vi "chopdata.vi"(8 "velo":dbl[][](array[numeric]), 9 "pos":dbl[](array[numeric])) -> (1 "slam_pos":dbl[](array[numeric]))   [LabVIEW 2012]
uses:
  G_SEN.vi
  <vilib>/Analysis/baseanly.llb/Real A x B.vi
  <vilib>/Analysis/7linalg.llb/Real SVD Decomposition.vi
  <vilib>/Analysis/Matrix/Numeric/Multiply/Multiply - RM,RM.vi
  <vilib>/Analysis/baseanly.llb/A x Vector.vi
  <vilib>/Analysis/Matrix/Numeric/Conversions/Matrix To Array - RM.vi
  <vilib>/Analysis/NI_AALBase.lvlib
  <vilib>/Analysis/NI_AALPro.lvlib
  <vilib>/Analysis/Matrix/NI_Matrix.lvlib
panel:
  out "y' 2":dbl
  in  "y 2":dbl
  in  "graph":bool
  out "iter 2":i32
  out "iter":i32
  out "error":dbl
  out "R'":dbl[][](array[numeric])
  out "y'":dbl
  out "x'":dbl
  out "mindata":dbl[][](array[numeric])
  out "keydata":dbl[][](array[numeric])
  out "zero_80_240":i32[][](array[numeric])
  out "time":u32
  out "x":dbl[](array[numeric])
  out "y":dbl[](array[numeric])
  out "XY Graph":cluster{"Y":dbl[], "Y":dbl[]}[](graph)
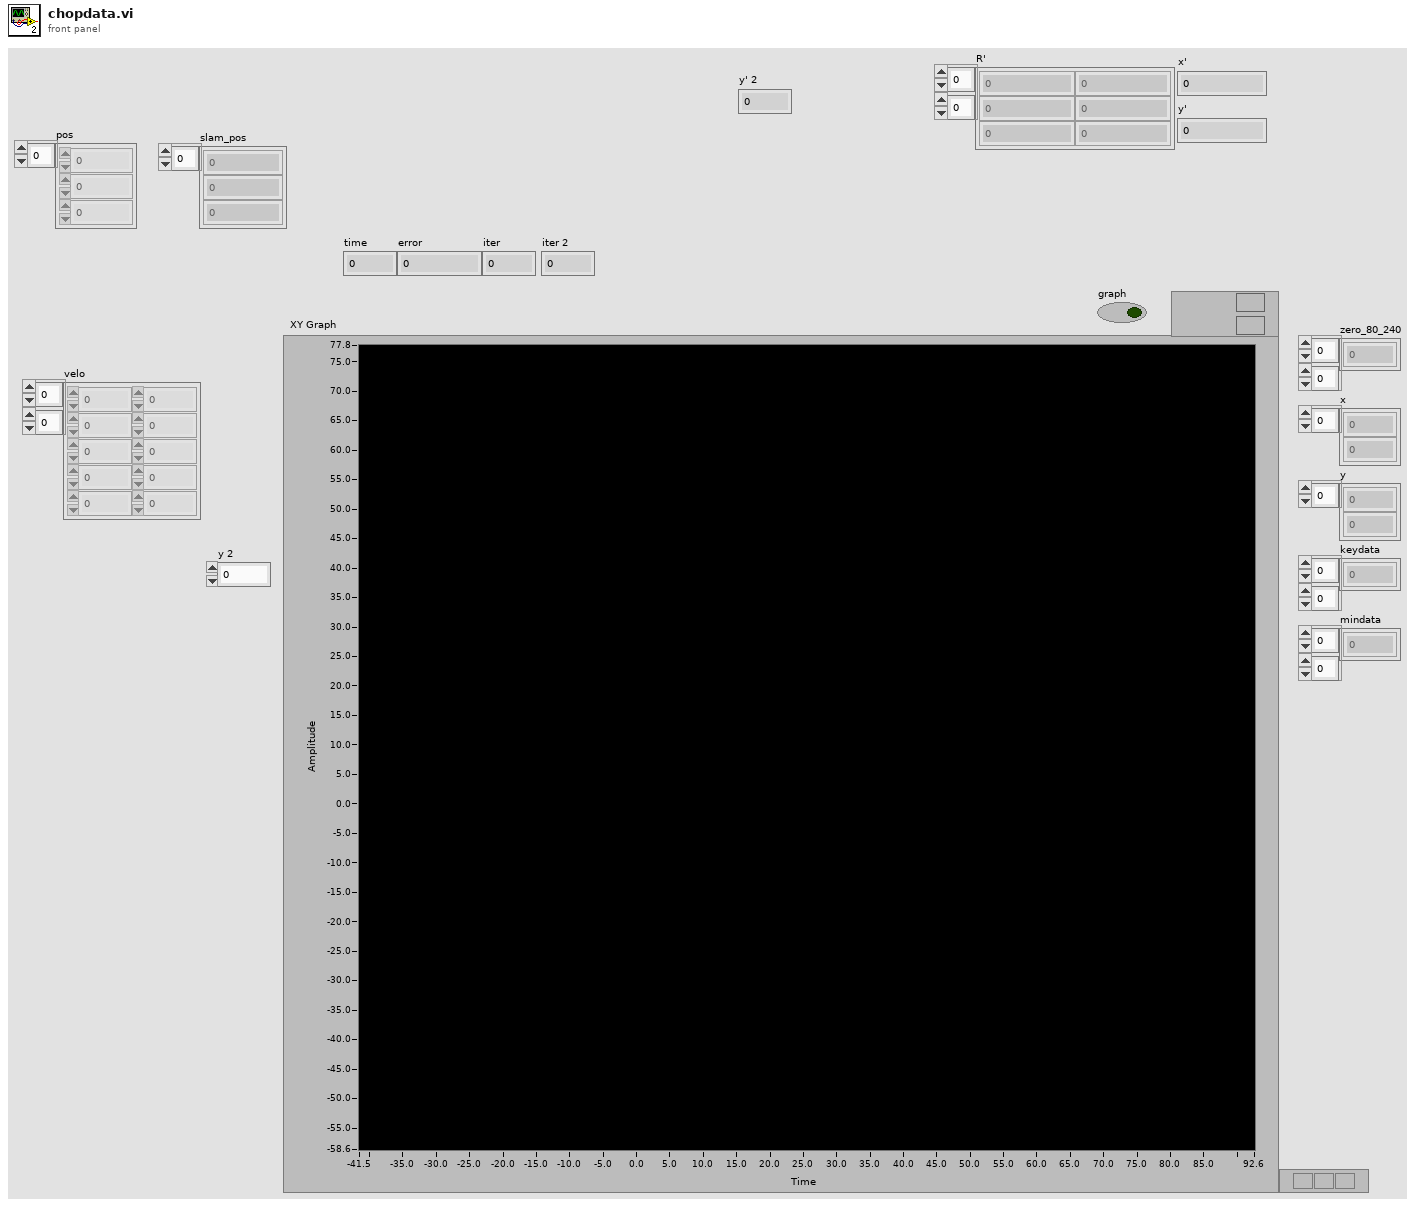
[diagram p1: front panel]
types:
  T1 = cluster{bool, "element":dbl, "element":dbl, "element":dbl}[]
  T2 = typedef "NI_Matrix.lvlib/RealMatrix.ctl" = dbl[][]
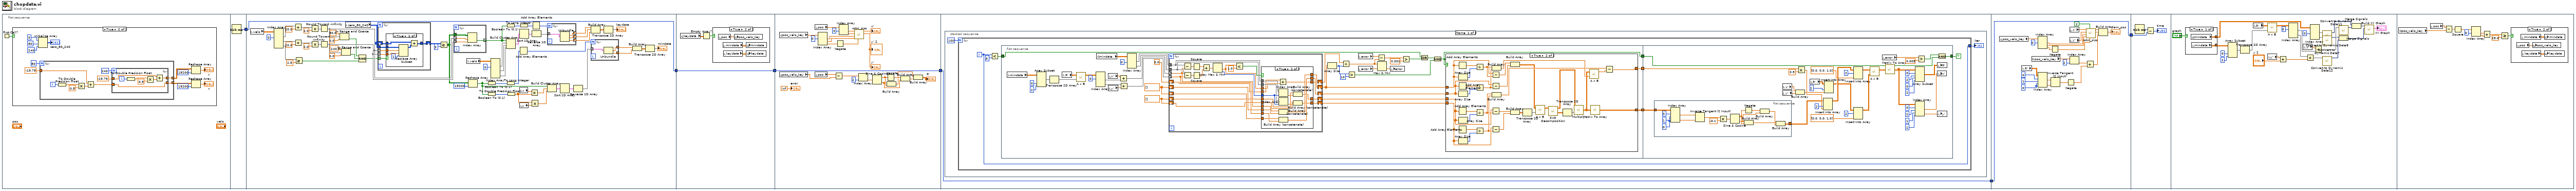
[diagram p0: block diagram]
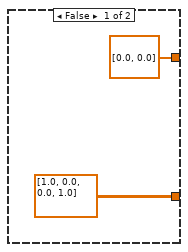
[diagram p5: hidden frame]
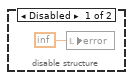
[diagram p8: hidden frame]
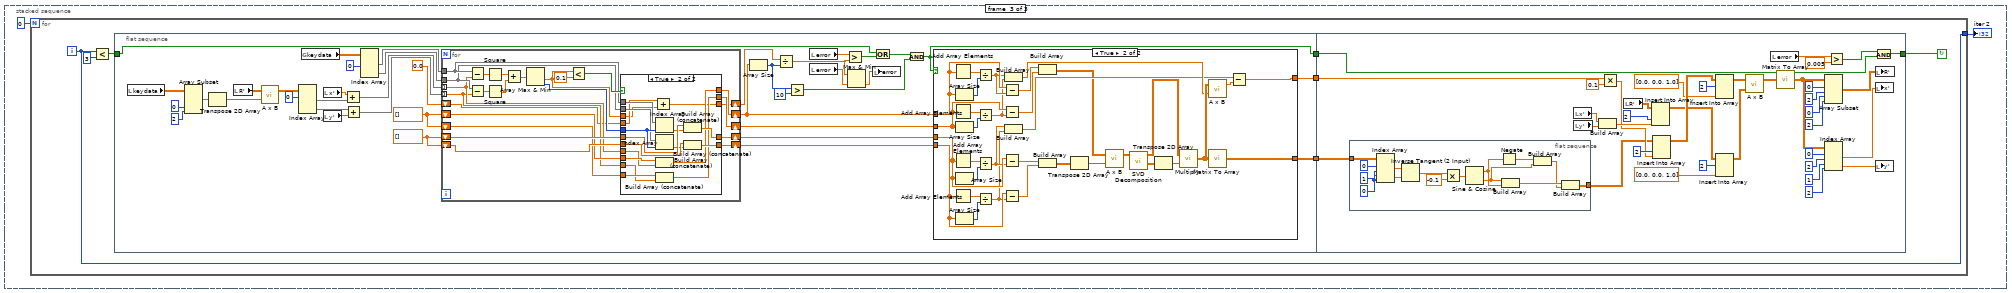
[diagram p9: hidden frame]
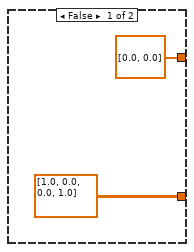
[diagram p10: hidden frame]
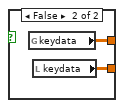
[diagram p12: hidden frame]
diagram:
  n1 = flat-sequence {
    tunnel: [w37] -> w6
    tunnel: w6 -> [w53]
    tunnel: [w53] -> w1
    tunnel: w1 -> [w129]
    tunnel: [w129] -> w5
    tunnel: w5 -> [w157]
    tunnel: [w157] -> w4
    tunnel: w4 -> [w158]
    tunnel: [w158] -> w3
    tunnel: w3 -> [w548]
    tunnel: [w548] -> w2
    tunnel: w2 -> [w550]
    frame #0 {
      n2 = First Call?() -> (First Call?: T/F=w7:bool)
      n3 = case shown="True" w7 {
        frame False {
        }
        frame True {
          n4 = Initialize Array(0, 80 ("dimension size"), 240 ("dimension size")) -> (→"zero_80_240":i32[][])
          n5 = for {
            N: 80 -> [_]
            tunnel: -19.75 -> [w27]
            tunnel: [w24] -> w12 mode=indexing
            tunnel: [w23] -> w17 mode=indexing
            i -> [w26]
            n6 = To Double Precision Float(number=w26) -> (double precision float=w22:dbl)
            n7 = Multiply(x=w22, y=0.5) -> (x*y=w20:dbl)
            n8 = Add(x=w27, y=w20) -> (x+y=w25:dbl)
            n9 = for {
              N: 240 -> [_]
              tunnel: -19.75 -> [w36]
              tunnel: [w34] -> w23 mode=indexing
              tunnel: w25 -> [w33]
              tunnel: [w33] -> w24 mode=indexing
              i -> [w35]
              n10 = To Double Precision Float(number=w35) -> (double precision float=w32:dbl)
              n11 = Multiply(x=w32, y=0.5) -> (x*y=w30:dbl)
              n12 = Add(x=w36, y=w30) -> (x+y=w34:dbl)
            }
          }
          n13 = Reshape Array(w17, 19200 ("dimension size")) -> (→"y":dbl[])
          n14 = Reshape Array(w12, 19200 ("dimension size")) -> (→"x":dbl[])
        }
      }
    }
    frame #1 {
      n15 = Tick Count (ms)() -> (millisecond timer value=w37:u32)
    }
    frame #2 {
      n16 = local read "velo"() -> (w48:dbl[][])
      n17 = Index Array(array=w48, index (col) #1=0 ("disabled index (col)")) -> (element #1=w78:dbl[], element #2=w77:dbl[], element #3=w40:dbl[])  [unwired: 5 in]
      n18 = Add(x=w78, y=20.0) -> (x+y=w74:dbl[])
      n19 = Add(x=w77, y=20.0) -> (x+y=w70:dbl[])
      n20 = Greater Or Equal?(x=w40, y=2.5) -> (x >= y?=w38:bool[])
      n21 = Multiply(x=w74, y=2.0) -> (x*y=w73:dbl[])
      n22 = Multiply(x=w70, y=2.0) -> (x*y=w69:dbl[])
      n23 = Round Toward -Infinity(1:w73) -> (0:w91:dbl[])
      n24 = Round Toward -Infinity(1:w69) -> (0:w92:dbl[])
      n25 = In Range and Coerce(upper limit=80.0, x=w91, lower limit=0.0) -> (In Range?=w86:bool[])  [unwired: 1 out]
      n26 = In Range and Coerce(upper limit=240.0, x=w92, lower limit=0.0) -> (In Range?=w87:bool[])  [unwired: 1 out]
      n27 = local read "zero_80_240"() -> (w52:i32[][])
      n28 = Compound Arithmetic op=AND(w86, w87, w38) -> (w88:bool[])
      n29 = for {
        shift-right: [w116] -> w90
        shift-left: w52 -> [w117]
        tunnel: w88 -> [w118] mode=indexing
        tunnel: w52 -> [w115]
        tunnel: w91 -> [w114] mode=indexing
        tunnel: w92 -> [w113] mode=indexing
        n30 = case shown="True" w118 {
          tunnel: w117 -> [w119 w122]
          tunnel: [w119 w120] -> w116
          tunnel: w115 -> [_ w126]
          tunnel: w114 -> [_ w125]
          tunnel: w113 -> [_ w124]
          frame False {
          }
          frame True {
            n31 = Replace Array Subset(array=w126, new element=1 ("new element/subarray"), index (row)=w125, index (col)=w124) -> (w121:i32[][])
            n32 = Add(x=w122, y=w121) -> (x+y=w120:i32[][])
          }
        }
      }
      n33 = Greater Or Equal?(x=w90, y=3) -> (x >= y?=w62:bool[][])
      n34 = for {
        tunnel: w62 -> [w112]
        tunnel: w91 -> [w111] mode=indexing
        tunnel: w92 -> [w110] mode=indexing
        tunnel: [w109] -> w95 mode=indexing
        n35 = Index Array(array=w112, index (row)=w111, index (col)=w110) -> (element=w109:bool)
      }
      n36 = local read "velo"() -> (w47:dbl[][])
      n37 = Reshape Array(w62, 19200 ("dimension size")) -> (w56:bool[])
      n38 = Boolean To (0,1)(Boolean=w56) -> (0, 1=w58:i16[])
      n39 = Boolean To (0,1)(Boolean=w56) -> (0, 1=w67:i16[])
      n40 = Index Array(array=w47, index (col) #1=0 ("disabled index (col)")) -> (element #1=w45:dbl[], element #2=w44:dbl[], element #3=w43:dbl[])  [unwired: 5 in]
      n41 = Boolean To (0,1)(Boolean=w95) -> (0, 1=w96:i16[])
      n42 = To Long Integer(number=w58) -> (32bit integer=w57:i32[])
      n43 = Build Cluster Array(w95, w45, w44, w43) -> (w93:T1)
      n44 = To Double Precision Float(number=w67) -> (double precision float=w61:dbl[])
      n45 = Add Array Elements(numeric array=w57) -> (sum=w55:i32)
      n46 = To Long Integer(number=w96) -> (32bit integer=w97:i32[])
      n47 = Sort 1D Array(array=w93) -> (sorted array=w94:T1)
      n48 = local read "x"() -> (w65:dbl[])
      n49 = local read "y"() -> (w66:dbl[])
      n50 = Multiply(x=w65, y=w61) -> (x*y=w64:dbl[])
      n51 = Multiply(x=w61, y=w66) -> (x*y=w63:dbl[])
      n52 = Add Array Elements(numeric array=w97) -> (sum=w98:i32)
      n53 = Reverse 1D Array(array=w94) -> (reversed array=w99:T1)
      n54 = for {
        N: w98 -> [_]
        tunnel: w99 -> [w108] mode=indexing
        tunnel: [w107] -> w76 mode=indexing
        tunnel: [w106] -> w75 mode=indexing
        tunnel: [w105] -> w100 mode=indexing
        n55 = Unbundle(w108) -> ("element"=w107:dbl, "element"=w106:dbl, "element"=w105:dbl)  [unwired: 1 out]
      }
      n56 = Build Cluster Array(w56, w64, w63) -> (w59:cluster{bool, dbl, dbl}[])
      n57 = Sort 1D Array(array=w59) -> (sorted array=w60:cluster{bool, dbl, dbl}[])
      n58 = Reverse 1D Array(array=w60) -> (reversed array=w54:cluster{bool, dbl, dbl}[])
      n59 = Build Array(w76, w75, w100) -> (w101:dbl[][])
      n60 = for {
        N: w55 -> [_]
        tunnel: w54 -> [w104] mode=indexing
        tunnel: [w103] -> w51 mode=indexing
        tunnel: [w102] -> w50 mode=indexing
        n61 = Unbundle(w104) -> (w103:dbl, w102:dbl)  [unwired: 1 out]
      }
      n62 = Transpose 2D Array(2D array=w101) -> (transposed array=→"keydata":dbl[][])
      n63 = Build Array(w51, w50) -> (w49:dbl[][])
      n64 = Transpose 2D Array(2D array=w49) -> (transposed array=→"mindata":dbl[][])
    }
    frame #3 {
      n65 = global read "G_SEN.vi" "keydata"() -> (w127:dbl[][])
      n66 = Empty Array?(array=w127) -> (empty?=w128:bool)
      n67 = case shown="True" w128 {
        frame False {
        }
        frame True {
          n68 = local read "pos"() -> (w130:dbl[])
          n69 = local read "mindata"() -> (w131:dbl[][])
          n70 = local read "keydata"() -> (w132:dbl[][])
          n71 = global write "G_SEN.vi" "pos_velo_key"(w130) -> ()
          n72 = global write "G_SEN.vi" "mindata"(w131) -> ()
          n73 = global write "G_SEN.vi" "keydata"(w132) -> ()
        }
      }
    }
    frame #4 {
      n74 = global read "G_SEN.vi" "pos_velo_key"() -> (w156:dbl[])
      n75 = global read "G_SEN.vi" "pos_velo_key"() -> (w143:dbl[])
      n76 = local read "pos"() -> (w150:dbl[])
      n77 = local read "pos"() -> (w144:dbl[])
      n78 = Index Array(array=w156, index #1=0 ("index")) -> (element #1=w154:dbl, element #2=w153:dbl, element #3=w152:dbl)  [unwired: 2 in]
      n79 = Subtract(x=w144, y=w143) -> (x-y=w142:dbl[])
      n80 = Negate(x=w152) -> (-x=w151:dbl)
      n81 = Index Array(array=w150, index #1=0 ("index")) -> (element #1=w148:dbl, element #2=w147:dbl)  [unwired: 1 in]
      n82 = call "rotm_siso.vi"("angle[rad]"=w151, "y0"=w153, "x0"=w154, "y"=w147, "x"=w148) -> ("y'"=→"y'" →"y' 2":dbl, "x'"=→"x'":dbl)  [unwired: 5 in]
      n83 = Index Array(array=w142, index=2) -> (element=w133:dbl)
      n84 = Sine & Cosine(0:w133) -> (1:w140:dbl, 2:w138:dbl)
      n85 = Negate(x=w140) -> (-x=w139:dbl)
      n86 = Build Array(w138, w140) -> (w137:dbl[])
      n87 = Build Array(w139, w138) -> (w136:dbl[])
      n88 = Build Array(w137, w136) -> (→"R'":dbl[][])
      "error" <- inf
    }
    frame #5 {
      n89 = stacked-sequence {
        frame #0 {
          n90 = for {
            N: 100 -> [_]
            tunnel: [w164] -> w159
            i -> [w164]
            stop <- w161 continue-if-true
            n91 = Less?(x=w164, y=3) -> (x < y?=w162:bool)
            n92 = flat-sequence {
              tunnel: [w208] -> w167
              tunnel: [w207] -> w166
              tunnel: [w206] -> w165
              tunnel: w162 -> [w205]
              tunnel: w167 -> [w292]
              tunnel: w166 -> [w296]
              tunnel: w165 -> [w297]
              tunnel: [w291] -> w161
              frame #0 {
                w185 = dbl[] []
                w186 = dbl[] []
                n93 = local read "mindata"() -> (w202:dbl[][])
                n94 = Array Subset(array=w202, index (col)=0 ("index"), length (col)=2 ("length")) -> (w199:dbl[][])  [unwired: 2 in]
                n95 = Transpose 2D Array(2D array=w199) -> (transposed array=w190:dbl[][])
                n96 = local read "R'"() -> (w191:dbl[][])
                n97 = call-poly <vilib>:"A x B.vi"("B"=w190, "A"=w191) -> ("A x B"=w189:T2)  [unwired: 1 out]
                n98 = Index Array(array=w189, index (row) #1=0 ("index (row)")) -> (element #1=w188:dbl[], element #2=w187:dbl[])  [unwired: 3 in]
                n99 = global read "G_SEN.vi" "mindata"() -> (w197:dbl[][])
                n100 = local read "x'"() -> (w204:dbl)
                n101 = local read "y'"() -> (w203:dbl)
                n102 = Add(x=w204, y=w188) -> (x+y=w193:dbl[])
                n103 = Add(x=w187, y=w203) -> (x+y=w192:dbl[])
                n104 = Index Array(array=w197, index (col) #1=0 ("disabled index (col)")) -> (element #1=w195:dbl[], element #2=w194:dbl[])  [unwired: 3 in]
                n105 = for {
                  tunnel: w195 -> [w259]
                  tunnel: w194 -> [w254]
                  tunnel: w193 -> [w249] mode=indexing
                  tunnel: w192 -> [w248] mode=indexing
                  shift-right: [w257] -> w180
                  shift-left: w186 -> [w260]
                  shift-right: [w255] -> w184
                  shift-left: w186 -> [w256]
                  shift-right: [w252] -> w176
                  shift-left: w185 -> [w253]
                  shift-right: [w250] -> w182
                  shift-left: w185 -> [w251]
                  shift-right: [w245] -> w179
                  shift-left: 0.0 -> [w247]
                  n106 = Subtract(x=w259, y=w249) -> (x-y=w266:dbl[])
                  n107 = Subtract(x=w254, y=w248) -> (x-y=w265:dbl[])
                  n108 = Square(x=w266) -> (x^2=w264:dbl[])
                  n109 = Square(x=w265) -> (x^2=w263:dbl[])
                  n110 = Add(x=w264, y=w263) -> (x+y=w262:dbl[])
                  n111 = Array Max & Min(array=w262) -> (min value=w246:dbl, min index (indices)=w258:i32)  [unwired: 2 out]
                  n112 = Less?(x=w246, y=1.0) -> (x < y?=w261:bool)
                  n113 = case shown="True" w261 {
                    tunnel: w260 -> [w271 w289]
                    tunnel: w259 -> [_ w288]
                    tunnel: w258 -> [_ w283]
                    tunnel: [w271 w286] -> w257
                    tunnel: w256 -> [w270 w285]
                    tunnel: [w270 w284] -> w255
                    tunnel: w254 -> [_ w282]
                    tunnel: w253 -> [w268 w280]
                    tunnel: [w268 w279] -> w252
                    tunnel: w251 -> [w269 w278]
                    tunnel: [w269 w277] -> w250
                    tunnel: w249 -> [_ w276]
                    tunnel: w248 -> [_ w275]
                    tunnel: w247 -> [w267 w274]
                    tunnel: w246 -> [_ w273]
                    tunnel: [w267 w272] -> w245
                    frame False {
                    }
                    frame True {
                      n114 = Add(x=w274, y=w273) -> (x+y=w272:dbl)
                      n115 = Index Array(array=w288, index=w283) -> (element=w287:dbl)
                      n116 = Index Array(array=w282, index=w283) -> (element=w281:dbl)
                      n117 = Build Array (concatenate)(w280, w276) -> (w279:dbl[])
                      n118 = Build Array (concatenate)(w278, w275) -> (w277:dbl[])
                      n119 = Build Array (concatenate)(w289, w287) -> (w286:dbl[])
                      n120 = Build Array (concatenate)(w285, w281) -> (w284:dbl[])
                    }
                  }
                }
                n121 = Array Size(array=w176) -> (size(s)=w178:i32)
                n122 = Divide(x=w179, y=w178) -> (x/y=w171:dbl)
                n123 = Greater?(x=w178, y=10) -> (0:w175:bool)
                n124 = local read "error"() -> (w172:dbl)
                n125 = local read "error"() -> (w177:dbl)
                n126 = Subtract(x=w172, y=w171) -> (x-y=w170:dbl)
                n127 = Max & Min(x=w171, y=w177) -> (min(x,y)=w173:dbl)  [unwired: 1 out]
                n128 = local write "error"(w173) -> ()
                n129 = Greater?(x=w170, y=0.001) -> (0:w169:bool)
                n130 = Or(x=w205, y=w169) -> (x .or. y?=w174:bool)
                n131 = And(x=w174, y=w175) -> (x .and. y?=w208:bool)
                n132 = case shown="True" w208 {
                  tunnel: [dbl[][] [[1.0, 0.0], [0.0, 1.0]] w240] -> w207
                  tunnel: w180 -> [_ w236]
                  tunnel: w184 -> [_ w232]
                  tunnel: w182 -> [_ w228]
                  tunnel: w176 -> [_ w224]
                  tunnel: [dbl[] [0.0, 0.0] w214] -> w206
                  frame False {
                  }
                  frame True {
                    n133 = Add Array Elements(numeric array=w224) -> (sum=w225:dbl)
                    n134 = Add Array Elements(numeric array=w228) -> (sum=w230:dbl)
                    n135 = Add Array Elements(numeric array=w236) -> (sum=w238:dbl)
                    n136 = Add Array Elements(numeric array=w232) -> (sum=w233:dbl)
                    n137 = Array Size(array=w224) -> (size(s)=w226:i32)
                    n138 = Array Size(array=w228) -> (size(s)=w229:i32)
                    n139 = Array Size(array=w236) -> (size(s)=w237:i32)
                    n140 = Array Size(array=w232) -> (size(s)=w234:i32)
                    n141 = Divide(x=w225, y=w226) -> (x/y=w222:dbl)
                    n142 = Divide(x=w230, y=w229) -> (x/y=w221:dbl)
                    n143 = Divide(x=w238, y=w237) -> (x/y=w220:dbl)
                    n144 = Divide(x=w233, y=w234) -> (x/y=w219:dbl)
                    n145 = Subtract(x=w224, y=w222) -> (x-y=w223:dbl[])
                    n146 = Subtract(x=w228, y=w221) -> (x-y=w227:dbl[])
                    n147 = Subtract(x=w236, y=w220) -> (x-y=w235:dbl[])
                    n148 = Subtract(x=w232, y=w219) -> (x-y=w231:dbl[])
                    n149 = Build Array(w222, w221) -> (w217:dbl[])
                    n150 = Build Array(w220, w219) -> (w215:dbl[])
                    n151 = Build Array(w223, w227) -> (w211:dbl[][])
                    n152 = Build Array(w235, w231) -> (w213:dbl[][])
                    n153 = Transpose 2D Array(2D array=w213) -> (transposed array=w212:dbl[][])
                    n154 = call-poly <vilib>:"A x B.vi"("B"=w212, "A"=w211) -> ("A x B"=w239:T2)  [unwired: 1 out]
                    n155 = call-poly <vilib>:"SVD Decomposition.vi"("A"=w239) -> ("Matrix V"=w241:T2, "Matrix U"=w242:T2)  [unwired: 6 in, 3 out]
                    n156 = Transpose 2D Array(2D array=w241) -> (transposed array=w243:T2)
                    n157 = call-poly <vilib>:"Multiply.vi"("Real Matrix B"=w243, "Real Matrix A"=w242) -> ("A * B"=w218:T2)
                    n158 = call-poly <vilib>:"A x B.vi"("Vector"=w217, "A"=w218) -> ("A x Vector"=w216:dbl[])  [unwired: 1 out]
                    n159 = call-poly <vilib>:"Matrix To Array.vi"("Real Matrix"=w218) -> ("Real 2D Array"=w240:dbl[][])
                    n160 = Subtract(x=w215, y=w216) -> (x-y=w214:dbl[])
                  }
                }
              }
              frame #1 {
                n161 = flat-sequence {
                  tunnel: w296 -> [w336]
                  tunnel: [w327] -> w295
                  frame #0 {
                    w341 = 0 ("disabled index (col)")
                    n162 = Index Array(array=w336, index (row) #1=0 ("disabled index (row)"), index (col) #1=1 ("disabled index (col)"), index (row) #2=w341, index (col) #2=w341) -> (element #1=w337:dbl, element #2=w338:dbl)
                    n163 = Inverse Tangent (2 Input)(1:w338, 2:w337) -> (0:w335:dbl)
                    n164 = Multiply(x=w335, y=-0.1) -> (x*y=w328:dbl)
                    n165 = Sine & Cosine(0:w328) -> (1:w333:dbl, 2:w331:dbl)
                    n166 = Negate(x=w333) -> (-x=w332:dbl)
                    n167 = Build Array(w331, w333) -> (w330:dbl[])
                    n168 = Build Array(w332, w331) -> (w329:dbl[])
                    n169 = Build Array(w330, w329) -> (w327:dbl[][])
                  }
                }
                n170 = local read "x'"() -> (w316:dbl)
                n171 = local read "y'"() -> (w317:dbl)
                n172 = Build Array(w316, w317) -> (w315:dbl[])
                n173 = Multiply(x=w297, y=0.5) -> (x*y=w299:dbl[])
                n174 = local read "R'"() -> (w319:dbl[][])
                n175 = Insert Into Array(array=w295, index (col)=2 ("disabled index (col)"), new element=w299) -> (w325:dbl[][])  [unwired: 1 in]
                n176 = Insert Into Array(array=w319, index (col)=2 ("disabled index (col)"), new element=w315) -> (w320:dbl[][])  [unwired: 1 in]
                n177 = Insert Into Array(array=w325, index (row)=2, new element=dbl[] [0.0, 0.0, 1.0]) -> (w314:dbl[][])  [unwired: 1 in]
                n178 = Insert Into Array(array=w320, index (row)=2, new element=dbl[] [0.0, 0.0, 1.0]) -> (w313:dbl[][])  [unwired: 1 in]
                n179 = call-poly <vilib>:"A x B.vi"("B"=w313, "A"=w314) -> ("A x B"=w308:T2)  [unwired: 1 out]
                n180 = local read "error"() -> (w290:dbl)
                n181 = call-poly <vilib>:"Matrix To Array.vi"("Real Matrix"=w308) -> ("Real 2D Array"=w306:dbl[][])
                n182 = Array Subset(array=w306, index (row)=0 ("index"), length (row)=2 ("length"), index (col)=0 ("index"), length (col)=2 ("length")) -> (w307:dbl[][])
                n183 = Index Array(array=w306, index (row) #1=0 ("disabled index (row)"), index (col) #1=2 ("disabled index (col)"), index (row) #2=1 ("index (row)"), index (col) #2=2 ("disabled index (col)")) -> (element #1=w301:dbl, element #2=w300:dbl)
                n184 = Greater?(x=w290, y=0.005) -> (0:w293:bool)
                n185 = And(x=w293, y=w292) -> (x .and. y?=w291:bool)
                n186 = local write "R'"(w307) -> ()
                n187 = local write "x'"(w301) -> ()
                n188 = local write "y'"(w300) -> ()
              }
            }
          }
          "iter" <- w159
        }
        frame #1 {
          n189 = disable-structure shown="Enabled" {
            frame Disabled {
              n190 = local write "error"(inf) -> ()
            }
            frame Enabled {
            }
          }
        }
        frame #2 {
          n191 = for {
            N: 0 -> [_]
            tunnel: [w348] -> w343
            i -> [w348]
            stop <- w345 continue-if-true
            n192 = Less?(x=w348, y=3) -> (x < y?=w346:bool)
            n193 = flat-sequence {
              tunnel: [w390] -> w351
              tunnel: [w389] -> w350
              tunnel: [w388] -> w349
              tunnel: w346 -> [w387]
              tunnel: w351 -> [w473]
              tunnel: w350 -> [w478]
              tunnel: w349 -> [w479]
              tunnel: [w472] -> w345
              frame #0 {
                w367 = dbl[] []
                w368 = dbl[] []
                n194 = local read "keydata"() -> (w384:dbl[][])
                n195 = Array Subset(array=w384, index (col)=0 ("index"), length (col)=2 ("length")) -> (w381:dbl[][])  [unwired: 2 in]
                n196 = Transpose 2D Array(2D array=w381) -> (transposed array=w372:dbl[][])
                n197 = local read "R'"() -> (w373:dbl[][])
                n198 = call-poly <vilib>:"A x B.vi"("B"=w372, "A"=w373) -> ("A x B"=w371:T2)  [unwired: 1 out]
                n199 = Index Array(array=w371, index (row) #1=0 ("index (row)")) -> (element #1=w370:dbl[], element #2=w369:dbl[])  [unwired: 3 in]
                n200 = global read "G_SEN.vi" "keydata"() -> (w379:dbl[][])
                n201 = local read "x'"() -> (w386:dbl)
                n202 = local read "y'"() -> (w385:dbl)
                n203 = Add(x=w386, y=w370) -> (x+y=w375:dbl[])
                n204 = Add(x=w369, y=w385) -> (x+y=w374:dbl[])
                n205 = Index Array(array=w379, index (col) #1=0 ("disabled index (col)")) -> (element #1=w377:dbl[], element #2=w376:dbl[])  [unwired: 3 in]
                n206 = for {
                  tunnel: w377 -> [w441]
                  tunnel: w376 -> [w436]
                  tunnel: w375 -> [w431] mode=indexing
                  tunnel: w374 -> [w430] mode=indexing
                  shift-right: [w439] -> w361
                  shift-left: w368 -> [w442]
                  shift-right: [w437] -> w366
                  shift-left: w368 -> [w438]
                  shift-right: [w434] -> w355
                  shift-left: w367 -> [w435]
                  shift-right: [w432] -> w363
                  shift-left: w367 -> [w433]
                  shift-right: [w427] -> w360
                  shift-left: 0.0 -> [w429]
                  n207 = Subtract(x=w441, y=w431) -> (x-y=w448:dbl[])
                  n208 = Subtract(x=w436, y=w430) -> (x-y=w447:dbl[])
                  n209 = Square(x=w448) -> (x^2=w446:dbl[])
                  n210 = Square(x=w447) -> (x^2=w445:dbl[])
                  n211 = Add(x=w446, y=w445) -> (x+y=w444:dbl[])
                  n212 = Array Max & Min(array=w444) -> (min value=w428:dbl, min index (indices)=w440:i32)  [unwired: 2 out]
                  n213 = Less?(x=w428, y=0.1) -> (x < y?=w443:bool)
                  n214 = case shown="True" w443 {
                    tunnel: w442 -> [w453 w471]
                    tunnel: w441 -> [_ w470]
                    tunnel: w440 -> [_ w465]
                    tunnel: [w453 w468] -> w439
                    tunnel: w438 -> [w452 w467]
                    tunnel: [w452 w466] -> w437
                    tunnel: w436 -> [_ w464]
                    tunnel: w435 -> [w450 w462]
                    tunnel: [w450 w461] -> w434
                    tunnel: w433 -> [w451 w460]
                    tunnel: [w451 w459] -> w432
                    tunnel: w431 -> [_ w458]
                    tunnel: w430 -> [_ w457]
                    tunnel: w429 -> [w449 w456]
                    tunnel: w428 -> [_ w455]
                    tunnel: [w449 w454] -> w427
                    frame False {
                    }
                    frame True {
                      n215 = Add(x=w456, y=w455) -> (x+y=w454:dbl)
                      n216 = Index Array(array=w470, index=w465) -> (element=w469:dbl)
                      n217 = Index Array(array=w464, index=w465) -> (element=w463:dbl)
                      n218 = Build Array (concatenate)(w462, w458) -> (w461:dbl[])
                      n219 = Build Array (concatenate)(w460, w457) -> (w459:dbl[])
                      n220 = Build Array (concatenate)(w471, w469) -> (w468:dbl[])
                      n221 = Build Array (concatenate)(w467, w463) -> (w466:dbl[])
                    }
                  }
                }
                n222 = Array Size(array=w355) -> (size(s)=w359:i32)
                n223 = Divide(x=w360, y=w359) -> (x/y=w358:dbl)
                n224 = Greater?(x=w359, y=10) -> (0:w353:bool)
                n225 = local read "error"() -> (w364:dbl)
                n226 = local read "error"() -> (w357:dbl)
                n227 = Greater?(x=w364, y=w358) -> (0:w354:bool)
                n228 = Max & Min(x=w358, y=w357) -> (min(x,y)=w356:dbl)  [unwired: 1 out]
                n229 = local write "error"(w356) -> ()
                n230 = Or(x=w387, y=w354) -> (x .or. y?=w352:bool)
                n231 = And(x=w352, y=w353) -> (x .and. y?=w390:bool)
                n232 = case shown="True" w390 {
                  tunnel: [dbl[][] [[1.0, 0.0], [0.0, 1.0]] w422] -> w389
                  tunnel: w361 -> [_ w418]
                  tunnel: w366 -> [_ w414]
                  tunnel: w363 -> [_ w410]
                  tunnel: w355 -> [_ w406]
                  tunnel: [dbl[] [0.0, 0.0] w396] -> w388
                  frame False {
                  }
                  frame True {
                    n233 = Add Array Elements(numeric array=w406) -> (sum=w407:dbl)
                    n234 = Add Array Elements(numeric array=w410) -> (sum=w412:dbl)
                    n235 = Add Array Elements(numeric array=w418) -> (sum=w420:dbl)
                    n236 = Add Array Elements(numeric array=w414) -> (sum=w415:dbl)
                    n237 = Array Size(array=w406) -> (size(s)=w408:i32)
                    n238 = Array Size(array=w410) -> (size(s)=w411:i32)
                    n239 = Array Size(array=w418) -> (size(s)=w419:i32)
                    n240 = Array Size(array=w414) -> (size(s)=w416:i32)
                    n241 = Divide(x=w407, y=w408) -> (x/y=w404:dbl)
                    n242 = Divide(x=w412, y=w411) -> (x/y=w403:dbl)
                    n243 = Divide(x=w420, y=w419) -> (x/y=w402:dbl)
                    n244 = Divide(x=w415, y=w416) -> (x/y=w401:dbl)
                    n245 = Subtract(x=w406, y=w404) -> (x-y=w405:dbl[])
                    n246 = Subtract(x=w410, y=w403) -> (x-y=w409:dbl[])
                    n247 = Subtract(x=w418, y=w402) -> (x-y=w417:dbl[])
                    n248 = Subtract(x=w414, y=w401) -> (x-y=w413:dbl[])
                    n249 = Build Array(w404, w403) -> (w399:dbl[])
                    n250 = Build Array(w402, w401) -> (w397:dbl[])
                    n251 = Build Array(w405, w409) -> (w393:dbl[][])
                    n252 = Build Array(w417, w413) -> (w395:dbl[][])
                    n253 = Transpose 2D Array(2D array=w395) -> (transposed array=w394:dbl[][])
                    n254 = call-poly <vilib>:"A x B.vi"("B"=w394, "A"=w393) -> ("A x B"=w421:T2)  [unwired: 1 out]
                    n255 = call-poly <vilib>:"SVD Decomposition.vi"("A"=w421) -> ("Matrix V"=w423:T2, "Matrix U"=w424:T2)  [unwired: 6 in, 3 out]
                    n256 = Transpose 2D Array(2D array=w423) -> (transposed array=w425:T2)
                    n257 = call-poly <vilib>:"Multiply.vi"("Real Matrix B"=w425, "Real Matrix A"=w424) -> ("A * B"=w400:T2)
                    n258 = call-poly <vilib>:"A x B.vi"("Vector"=w399, "A"=w400) -> ("A x Vector"=w398:dbl[])  [unwired: 1 out]
                    n259 = call-poly <vilib>:"Matrix To Array.vi"("Real Matrix"=w400) -> ("Real 2D Array"=w422:dbl[][])
                    n260 = Subtract(x=w397, y=w398) -> (x-y=w396:dbl[])
                  }
                }
              }
              frame #1 {
                n261 = flat-sequence {
                  tunnel: w478 -> [w518]
                  tunnel: [w509] -> w477
                  frame #0 {
                    w523 = 0 ("disabled index (col)")
                    n262 = Index Array(array=w518, index (row) #1=0 ("disabled index (row)"), index (col) #1=1 ("disabled index (col)"), index (row) #2=w523, index (col) #2=w523) -> (element #1=w519:dbl, element #2=w520:dbl)
                    n263 = Inverse Tangent (2 Input)(1:w520, 2:w519) -> (0:w517:dbl)
                    n264 = Multiply(x=w517, y=-0.1) -> (x*y=w510:dbl)
                    n265 = Sine & Cosine(0:w510) -> (1:w515:dbl, 2:w513:dbl)
                    n266 = Negate(x=w515) -> (-x=w514:dbl)
                    n267 = Build Array(w513, w515) -> (w512:dbl[])
                    n268 = Build Array(w514, w513) -> (w511:dbl[])
                    n269 = Build Array(w512, w511) -> (w509:dbl[][])
                  }
                }
                n270 = local read "x'"() -> (w498:dbl)
                n271 = local read "y'"() -> (w499:dbl)
                n272 = Build Array(w498, w499) -> (w497:dbl[])
                n273 = Multiply(x=w479, y=0.1) -> (x*y=w481:dbl[])
                n274 = local read "R'"() -> (w501:dbl[][])
                n275 = Insert Into Array(array=w501, index (col)=2 ("disabled index (col)"), new element=w497) -> (w502:dbl[][])  [unwired: 1 in]
                n276 = Insert Into Array(array=w477, index (col)=2 ("disabled index (col)"), new element=w481) -> (w507:dbl[][])  [unwired: 1 in]
                n277 = Insert Into Array(array=w507, index (row)=2, new element=dbl[] [0.0, 0.0, 1.0]) -> (w496:dbl[][])  [unwired: 1 in]
                n278 = Insert Into Array(array=w502, index (row)=2, new element=dbl[] [0.0, 0.0, 1.0]) -> (w495:dbl[][])  [unwired: 1 in]
                n279 = call-poly <vilib>:"A x B.vi"("B"=w495, "A"=w496) -> ("A x B"=w490:T2)  [unwired: 1 out]
                n280 = local read "error"() -> (w475:dbl)
                n281 = call-poly <vilib>:"Matrix To Array.vi"("Real Matrix"=w490) -> ("Real 2D Array"=w488:dbl[][])
                n282 = Array Subset(array=w488, index (row)=0 ("index"), length (row)=2 ("length"), index (col)=0 ("index"), length (col)=2 ("length")) -> (w489:dbl[][])
                n283 = Index Array(array=w488, index (row) #1=0 ("disabled index (row)"), index (col) #1=2 ("disabled index (col)"), index (row) #2=1 ("index (row)"), index (col) #2=2 ("disabled index (col)")) -> (element #1=w483:dbl, element #2=w482:dbl)
                n284 = Greater?(x=w475, y=0.005) -> (0:w474:bool)
                n285 = And(x=w474, y=w473) -> (x .and. y?=w472:bool)
                n286 = local write "R'"(w489) -> ()
                n287 = local write "x'"(w483) -> ()
                n288 = local write "y'"(w482) -> ()
              }
            }
          }
          "iter 2" <- w343
        }
      }
    }
    frame #6 {
      w543 = 0 ("disabled index (col)")
      n289 = global read "G_SEN.vi" "pos_velo_key"() -> (w538:dbl[])
      n290 = local read "R'"() -> (w542:dbl[][])
      n291 = global read "G_SEN.vi" "pos_velo_key"() -> (w541:dbl[])
      n292 = Index Array(array=w538, index #1=0 ("index")) -> (element #1=w536:dbl, element #2=w535:dbl, element #3=w534:dbl)  [unwired: 2 in]
      n293 = Index Array(array=w542, index (row) #1=0 ("disabled index (row)"), index (col) #1=1 ("disabled index (col)"), index (row) #2=w543, index (col) #2=w543) -> (element #1=w547:dbl, element #2=w546:dbl)
      n294 = Negate(x=w534) -> (-x=w533:dbl)
      n295 = Inverse Tangent (2 Input)(1:w546, 2:w547) -> (0:w525:dbl)
      n296 = Negate(x=w525) -> (-x=w524:dbl)
      n297 = local read "x'"() -> (w532:dbl)
      n298 = local read "y'"() -> (w531:dbl)
      n299 = Index Array(array=w541, index=2) -> (element=w539:dbl)
      n300 = Add(x=w539, y=w524) -> (x+y=w527:dbl)
      n301 = call "rotm_siso.vi"("angle[rad]"=w533, "reverse"=TRUE, "y0"=w535, "x0"=w536, "y"=w531, "x"=w532) -> ("y'"=w528:dbl, "x'"=w529:dbl)  [unwired: 4 in]
      n302 = Build Array(w529, w528, w527) -> (→"slam_pos":dbl[])
    }
    frame #7 {
      n303 = Tick Count (ms)() -> (millisecond timer value=w551:u32)
      n304 = Subtract(x=w551, y=w550) -> (x-y=→"time":u32)
    }
    frame #8 {
      n305 = case shown="True" "graph" {
        tunnel: [w581 w583] -> w575
        tunnel: [w580 w582] -> w568
        frame True {
          n306 = global read "G_SEN.vi" "mindata"() -> (w581:dbl[][])
          n307 = local read "mindata"() -> (w580:dbl[][])
        }
        frame False {
          n308 = global read "G_SEN.vi" "keydata"() -> (w583:dbl[][])
          n309 = local read "keydata"() -> (w582:dbl[][])
        }
      }
      n310 = Array Subset(array=w568, index (col)=0 ("index"), length (col)=2 ("length")) -> (w565:dbl[][])  [unwired: 2 in]
      n311 = Transpose 2D Array(2D array=w565) -> (transposed array=w564:dbl[][])
      n312 = local read "R'"() -> (w569:dbl[][])
      n313 = call-poly <vilib>:"A x B.vi"("B"=w564, "A"=w569) -> ("A x B"=w563:T2)  [unwired: 1 out]
      n314 = local read "y'"() -> (w554:dbl)
      n315 = Add(x=w554, y="y 2") -> (x+y=w553:dbl)
      n316 = Index Array(array=w563, index (row) #1=0 ("index (row)")) -> (element #1=w573:dbl[], element #2=w572:dbl[])  [unwired: 3 in]
      n317 = local read "x'"() -> (w574:dbl)
      n318 = Add(x=w572, y=w553) -> (x+y=w570:dbl[])
      n319 = Index Array(array=w575, index (col) #1=0 ("disabled index (col)")) -> (element #1=w577:dbl[], element #2=w578:dbl[])  [unwired: 3 in]
      n320 = Add(x=w574, y=w573) -> (x+y=w571:dbl[])
      n321 = call "Convert to Dynamic Data8"("Array"=w577) -> ("Dynamic Data Type"=w561:dynamicdata)  [unwired: 3 in]
      n322 = call "Convert to Dynamic Data7"("Array"=w578) -> ("Dynamic Data Type"=w558:dynamicdata)  [unwired: 3 in]
      n323 = call "Convert to Dynamic Data12"("Array"=w570) -> ("Dynamic Data Type"=w556:dynamicdata)  [unwired: 3 in]
      n324 = call "Convert to Dynamic Data11"("Array"=w571) -> ("Dynamic Data Type"=w559:dynamicdata)  [unwired: 3 in]
      n325 = Merge Signals(w558, w556) -> (w557:dynamicdata)
      n326 = Merge Signals(w561, w559) -> (w560:dynamicdata)
      n327 = call "Build XY Graph"("Y Input"=w557, "X Input"=w560) -> ("XY Graph"=→"XY Graph":cluster{"Y":dbl[], "Y":dbl[]}[])  [unwired: 3 in, 6 out]
    }
    frame #9 {
      n328 = global read "G_SEN.vi" "pos_velo_key"() -> (w585:dbl[])
      n329 = local read "pos"() -> (w584:dbl[])
      n330 = Subtract(x=w584, y=w585) -> (x-y=w586:dbl[])
      n331 = Square(x=w586) -> (x^2=w587:dbl[])
      n332 = Index Array(array=w587, index #1=0 ("index")) -> (element #1=w589:dbl, element #2=w590:dbl)  [unwired: 1 in]
      n333 = Add(x=w589, y=w590) -> (x+y=w591:dbl)
      n334 = Greater Or Equal?(x=w591, y=25.0) -> (x >= y?=w593:bool)
      n335 = case shown="True" w593 {
        frame False {
        }
        frame True {
          n336 = local read "pos"() -> (w594:dbl[])
          n337 = local read "mindata"() -> (w595:dbl[][])
          n338 = local read "keydata"() -> (w596:dbl[][])
          n339 = global write "G_SEN.vi" "pos_velo_key"(w594) -> ()
          n340 = global write "G_SEN.vi" "mindata"(w595) -> ()
          n341 = global write "G_SEN.vi" "keydata"(w596) -> ()
        }
      }
    }
  }
